vi "List Classes and Interfaces.vi"(11 "error in (no error)":errorcluster) -> (4 "Class Names":string[](array[string]), 6 "Class Paths":path[](array[path]), 8 "Interface Names":string[](array[string]), 10 "Interface Paths":path[](array[path]), 15 "error out":errorcluster)   [LabVIEW 2019, in "ClassLoader.lvlib"]
doc: "List all cached class names and paths separated into class and interface arrays.\n\nThis VI does not automatically load data. Front-load before calling this VI!"
uses:
  ClassLoader.lvlib
  Sub/Cache/Cache_Path Global.vi
  Sub/Cache/Cache_Info Global.vi
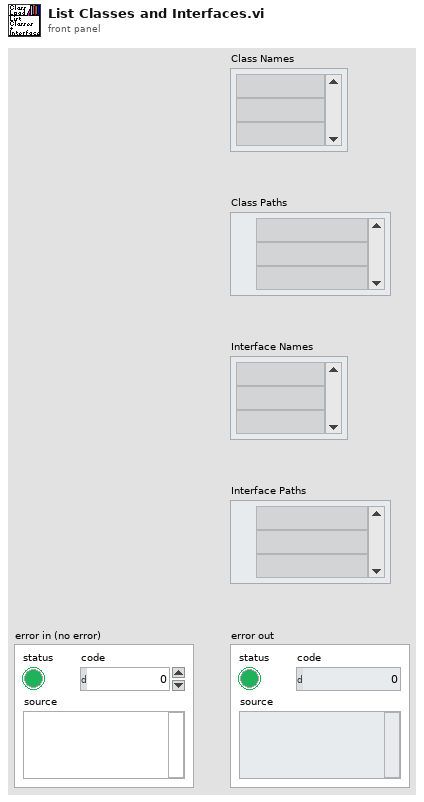
[diagram p1: front panel]
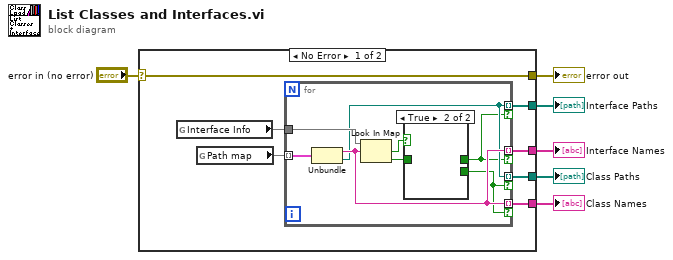
[diagram p0: block diagram]
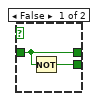
[diagram p2: hidden frame]
diagram:
  n1 = case shown="No Error" "error in (no error)" {
    selector: "error in (no error)" -> [w10 w24]
    tunnel: [w12 _] -> w6
    tunnel: [w11 _] -> w5
    tunnel: [w10 w24] -> w3
    tunnel: [w8 _] -> w2
    tunnel: [w7 _] -> w1
    frame No Error {
      n2 = global read "Cache_Info Global.vi" "Interface Info"() -> (w9:map{string, bool})
      n3 = global read "Cache_Path Global.vi" "Path map"() -> (w13:map{string, path})
      n4 = for {
        tunnel: w13 -> [w21] mode=indexing
        tunnel: [w19] -> w12 mode=indexing if=w15
        tunnel: [w18] -> w11 mode=indexing if=w15
        tunnel: w9 -> [w20]
        tunnel: [w19] -> w8 mode=indexing if=w14
        tunnel: [w18] -> w7 mode=indexing if=w14
        n5 = Unbundle(w21) -> ("key"=w19:string, "value"=w18:path)
        n6 = Look In Map(map=w20, key=w19) -> (key not found?=w17:bool, value=w16:bool)  [unwired: 1 in]
        n7 = case shown="True" w17 {
          tunnel: w16 -> [w22 _]
          tunnel: [w23 _] -> w15
          tunnel: [w22 _] -> w14
          frame False {
            n8 = Not(x=w22) -> (.not. x?=w23:bool)
          }
          frame True {
          }
        }
      }
    }
    frame Error {
    }
  }
  "error out" <- w3
  "Class Paths" <- w5
  "Class Names" <- w6
  "Interface Paths" <- w1
  "Interface Names" <- w2
